vi "App_User Registering.vi"() -> ()   [LabVIEW 2015, in "Application 1.lvlib"]
uses:
  Application 1.lvlib
panel:
  in  "Registering":bool caption="Blank"
  in  "Phone Number":string caption="String"
  in  "Email":string caption="String"
  in  "User Name":string caption="String"
  in  "Open Image":bool
  in  "Snap":bool
  out "User Picture":T1(plugin-control)
  # "*"
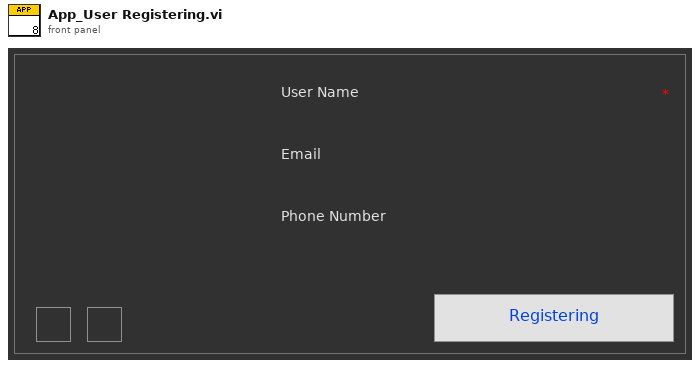
[diagram p1: front panel]
types:
  T1 = typedef "IMAQ Image.ctl" = refnum<image>
  T2 = typedef "Image Type" = u32
  T3 = cluster{"Image Out":T1, "User Name":string, "Email":string, "Phone Number":string}
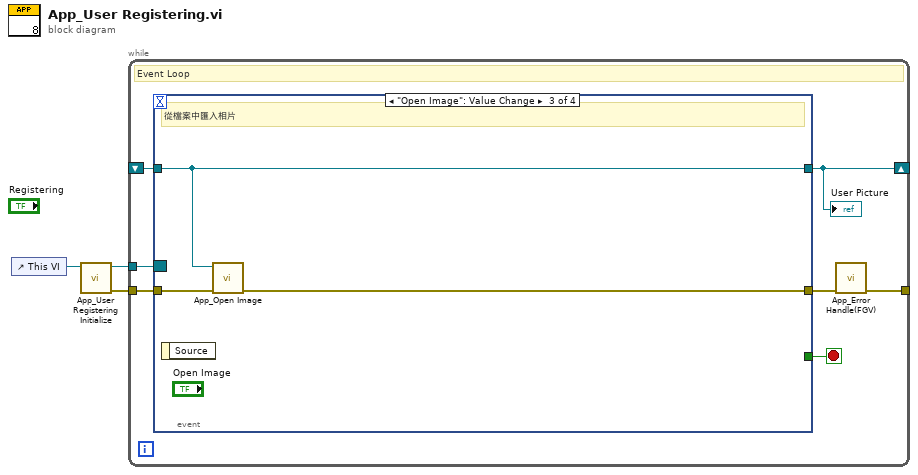
[diagram p0: block diagram]
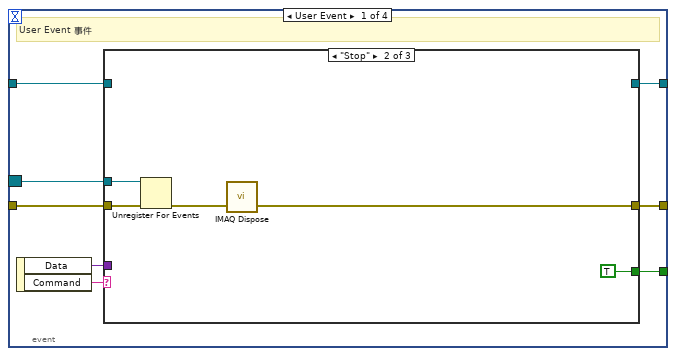
[diagram p2: hidden frame]
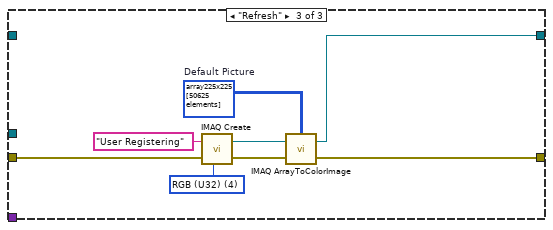
[diagram p4: hidden frame]
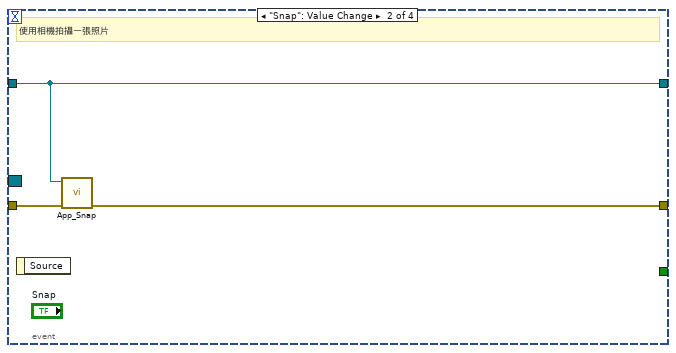
[diagram p5: hidden frame]
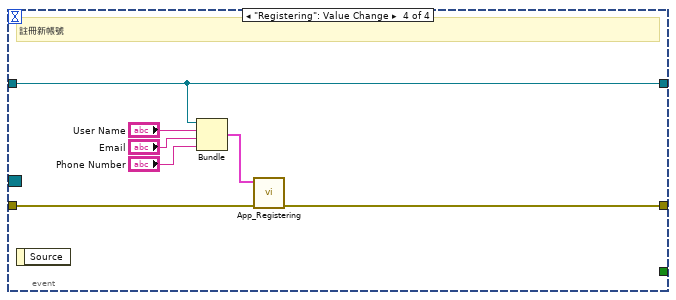
[diagram p6: hidden frame]
diagram:
  n1 = control-ref of="This VI"() -> (w3:refnum<vi>)
  n2 = call "App_User Registering Initialize.vi"("VI Reference"=w3) -> ("error out"=w1:errorcluster, "Event Registration Refnum"=w2:refnum<event-registration>)  [unwired: 9 in]
  n3 = while {
    tunnel: w2 -> [w10]
    tunnel: w1 -> [w9]
    shift-right: [w4] -> _
    shift-left: _ -> [w7]
    tunnel: [w5] -> _
    stop <- w8 stop-if-true
    # "Event Loop"
    n4 = event shown="[2] \"Open Image\": Value Change" {
      selector: w10 -> [w15 _ _ _]
      dyn-events: _ -> [_ _ _ _]
      timeout: _ -> [_ _ _ _]
      tunnel: w9 -> [w16 w36 w39 w42]
      tunnel: [w14 w34 w38 w40] -> w6
      tunnel: [w13 _ _ _] -> w8
      tunnel: [w12 w35 w37 w44] -> w4
      tunnel: w7 -> [w11 w35 w37 w44]
      event User Event {
        # "User Event 事件"
        n5 = event-data() -> ("Data"=w17:variant, "Command"=w18:string)  [unwired: 1 in]
        n6 = case shown="\"Stop\"" w18 {
          tunnel: w17 -> [_ _ _]
          tunnel: w16 -> [w20 w25 w33]
          tunnel: w15 -> [_ w24 _]
          tunnel: [w20 w21 w26] -> w14
          tunnel: [_ TRUE _] -> w13
          tunnel: [w19 _ w27] -> w12
          tunnel: w11 -> [w19 _ _]
          frame Default {
          }
          frame "Stop" {
            n7 = Unregister For Events(event registration refnum=w24, error in=w25) -> (error out=w22:errorcluster)
            n8 = call "IMAQ Dispose"("error in (no error)"=w22) -> ("error out"=w21:errorcluster)  [unwired: 5 in]
          }
          frame "Refresh" {
            w28 = u32[][] array225x225[50625 elements]  # Default Picture
            w31 = T2 4 items=["Grayscale (U8)", "Grayscale (I16)", "Grayscale (SGL)", "Complex (CSG)", "RGB (U32)", "HSL (U32)", "RGB (U64)", "Grayscale (U16)"] ("Image Type")
            n9 = call "IMAQ Create"("Image Name"="User Registering", "Image Type"=w31, "error in (no error)"=w33) -> ("New Image"=w29:T1, "error out"=w30:errorcluster)  [unwired: 2 in]
            n10 = call "IMAQ ArrayToColorImage"("Image Pixels (U32)"=w28, "Image"=w29, "error in (no error)"=w30) -> ("Image Out"=w27:T1, "error out"=w26:errorcluster)  [unwired: 2 in]
          }
        }
      }
      event "Snap": Value Change {
        # "使用相機拍攝一張照片"
        n11 = event-data() -> ()  [unwired: 1 in, 1 out]
        n12 = call "App_Snap.vi"("error in"=w36, "Image"=w35) -> ("error out"=w34:errorcluster)  [unwired: 9 in]
      }
      event "Open Image": Value Change {
        # "從檔案中匯入相片"
        n13 = event-data() -> ()  [unwired: 1 in, 1 out]
        n14 = call "App_Open Image.vi"("error in"=w39, "Image"=w37) -> ("error out"=w38:errorcluster)  [unwired: 9 in]
      }
      event "Registering": Value Change {
        # "註冊新帳號"
        n15 = event-data() -> ()  [unwired: 1 in, 1 out]
        n16 = Bundle("Image Out"=w44, "User Name"="User Name", "Email"="Email", "Phone Number"="Phone Number") -> (w41:T3)  [unwired: 1 in]
        n17 = call "App_Registering.vi"("error in"=w42, "Registering Data"=w41) -> ("error out"=w40:errorcluster)  [unwired: 9 in]
      }
    }
    "User Picture" <- w4
    n18 = call "App_Error Handle(FGV).vi"("error in"=w6) -> ("error out"=w5:errorcluster)  [unwired: 9 in, 1 out]
  }
